vi "Sample Application.vi"() -> ()   [LabVIEW 2010]
doc: "This is a demo to understand how to use Solo Server and Instant PLUS for online license activation."
uses:
  C:/Program Files (x86)/SoftwareKey/Instant PLUS/IP2Lib32.dll
panel:
  in  "Upgrade to Ultimate":bool
  in  "Exit":bool
  in  "Deactviate":bool
  out "Activated Version":bool
  out "Demo  Version":bool
  out "AW Ultimate Mode":bool
  out "AW Ultra Mode":bool
  out "AW Omnia Mode":bool
  # "Sample Application"
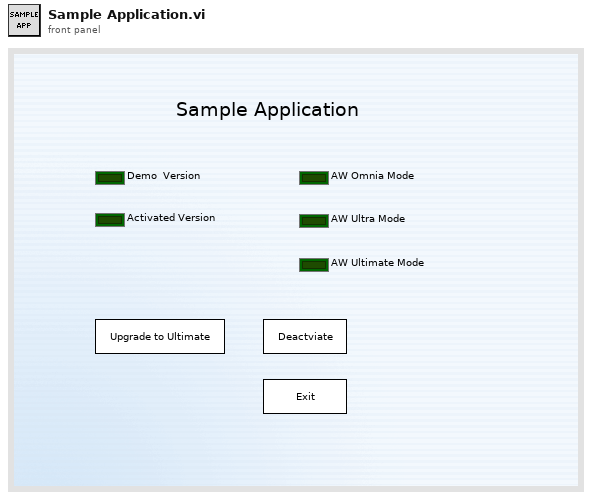
[diagram p1: front panel]
types:
  T1 = enum8{"Enabled", "Disabled", "Disabled and Grayed Out"}
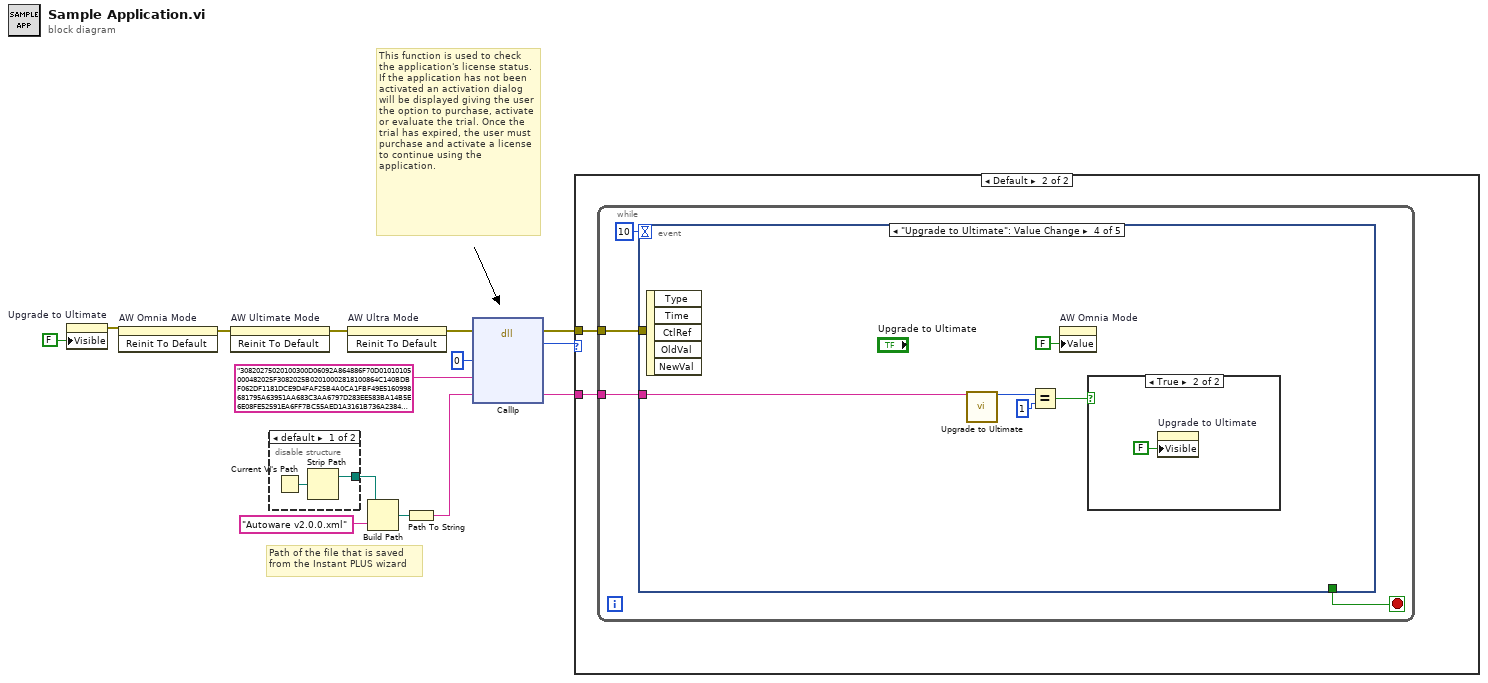
[diagram p0: block diagram]
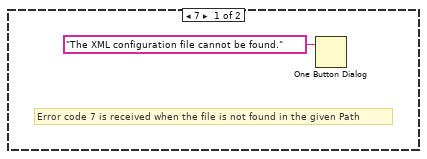
[diagram p2: hidden frame]
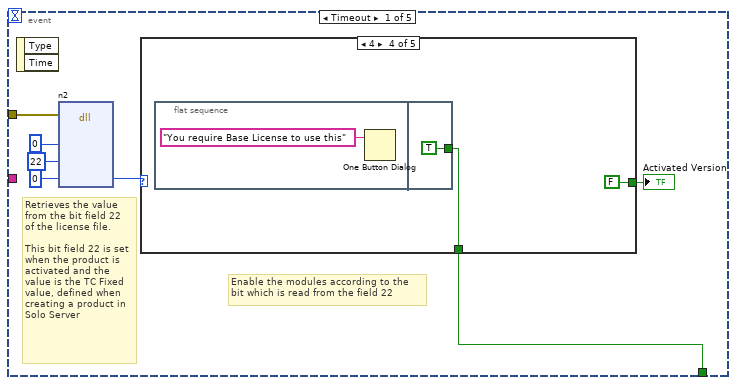
[diagram p3: hidden frame]
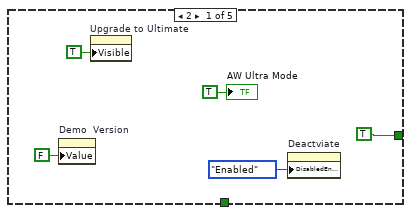
[diagram p4: hidden frame]
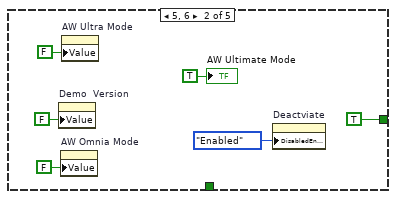
[diagram p5: hidden frame]
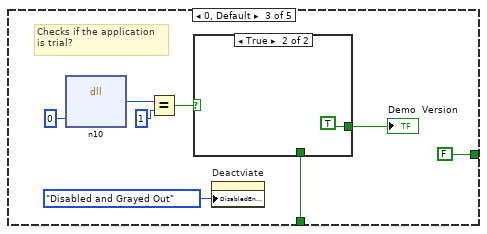
[diagram p6: hidden frame]
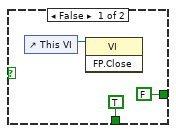
[diagram p7: hidden frame]
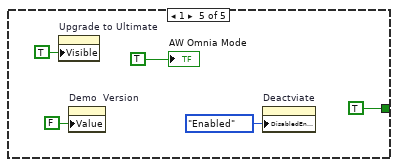
[diagram p8: hidden frame]
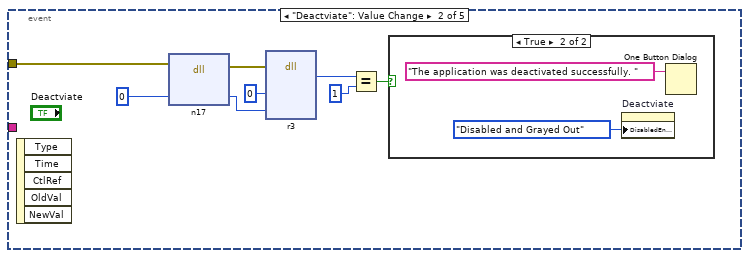
[diagram p9: hidden frame]
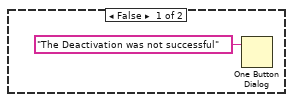
[diagram p10: hidden frame]
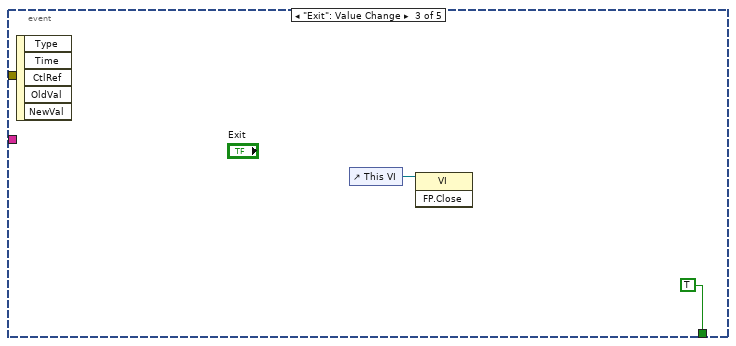
[diagram p11: hidden frame]
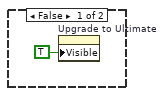
[diagram p12: hidden frame]
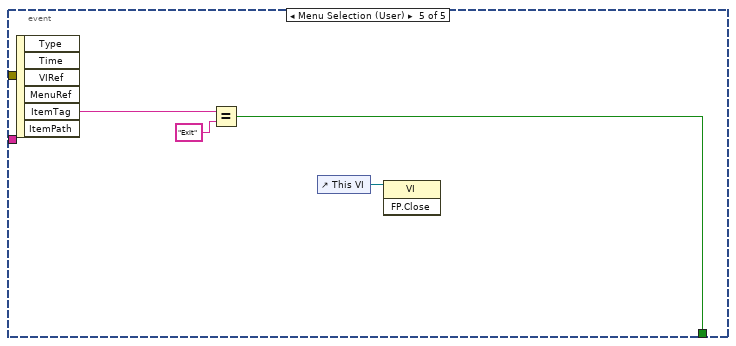
[diagram p13: hidden frame]
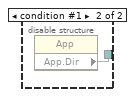
[diagram p14: hidden frame]
diagram:
  # "Path of the file that is saved \nfrom the Instant PLUS wizard"
  # "This function is used to check the application's license status. If the application has not been activated an activation dialog will be displayed giving the user the option to purchase, activate or evaluate the trial. Once the trial has expired, the user must purchase and activate a license to continue using the application."
  n1 = property on="Upgrade to Ultimate" class="Bool"("Visible"=FALSE) -> (error out=w3:errorcluster)  [unwired: 2 in, 1 out]
  n2 = invoke on="AW Omnia Mode" class="Bool (strict)" method="Reinit To Default"(error in=w3) -> (error out=w9:errorcluster)  [unwired: 2 in, 2 out]
  n3 = invoke on="AW Ultimate Mode" class="Bool (strict)" method="Reinit To Default"(error in=w9) -> (error out=w8:errorcluster)  [unwired: 2 in, 2 out]
  n4 = disable-structure shown="default" {
    disable-tunnel: [w16 w17] -> w2
    frame condition #0 (active) {
      n5 = Current VI's Path() -> (path=w15:path)
      n6 = Strip Path(path=w15) -> (stripped path=w16:path)  [unwired: 1 out]
    }
    frame condition #1 {
      n7 = property class="App"() -> ("App.Dir"=w17:path)  [unwired: 2 in, 2 out]
    }
  }
  n8 = invoke on="AW Ultra Mode" class="Bool (strict)" method="Reinit To Default"(error in=w8) -> (error out=w7:errorcluster)  [unwired: 2 in, 2 out]
  n9 = Build Path(base path=w2, name or relative path="Autoware v2.0.0.xml") -> (appended path=w13:path)
  n10 = Path To String(path=w13) -> (string=w14:string)
  n11 = dll-call lib="C:/Program Files (x86)/SoftwareKey/Instant PLUS/IP2Lib32.dll" fn="CallIp"(error in=w7, "flags"=0, "key"="30820275020100300D06092A864886F70D01010105000482025F3082025B02010002818100864C140BDBF062DF1181DCE9D4FAF25B4A0CA1FBF49E5160998681795A63951AA683C3AA6797D283EE583BA14B5E6E08FE52591EA6FF7BC55AED1A3161B736A2384D870C7207CC8E0C44F3FA09198B5C5B93A3664E7E03A0649458AD77C39D105654BF6D9AB9740C204A6EEE81CCFF07CA72CE9B1B6C7B6A51E0E7FB828A71050201110281802B72F76D3FA09875587CD687E305E4FF6AC7DA0DC0151A53F56F48019D3E55E2F9A319A81274E239BE0D7CB42EF8E75D4338C27ADBAD02657F4CB5A6908E193403A635934E3586225F27BF45D9C9E9ED9CFCFD5F08C52C6CFB1FB7415746DD7D51C4C534D770EAAE174BC1FFC315035FFAA70DEA8A613053DEEFD2921B82A04302...", "path"=w14) -> (error out=w5:errorcluster, "result"=w6:i32, "path"=w1:string)  [unwired: 4 in, 1 out]
  n12 = case shown="Default" w6 {
    tunnel: w5 -> [_ w20]
    tunnel: w1 -> [_ w19]
    frame 7 {
      # "Error code 7 is received when the file is not found in the given Path"
      n13 = One Button Dialog(message="The XML configuration file cannot be found.") -> ()  [unwired: 1 in, 1 out]
    }
    frame Default {
      n14 = while {
        tunnel: w20 -> [w22]
        tunnel: w19 -> [w21]
        stop <- w23 stop-if-true
        n15 = event shown="[3] \"Upgrade to Ultimate\": Value Change" {
          selector: _ -> [_ _ _ _ _]
          dyn-events: _ -> [_ _ _ _ _]
          timeout: 10 -> [_ _ _ _ _]
          tunnel: [w30 _ TRUE ("Exit") _ w85] -> w23
          tunnel: w22 -> [w25 w67 _ _ _]
          tunnel: w21 -> [_ _ _ w77 _]
          event Timeout {
            # "Enable the modules according to the\nbit which is read from the field 22"
            # "Retrieves the value\nfrom the bit field 22\nof the license file.\n\nThis bit field 22 is set\nwhen the product is \nactivated and the \nvalue is the TC Fixed \nvalue, defined when\ncreating a product in\nSolo Server"
            n16 = event-data() -> ()  [unwired: 1 in, 2 out]
            n17 = dll-call lib="C:/Program Files (x86)/SoftwareKey/Instant PLUS/IP2Lib32.dll" fn="n2"(error in=w25, "flags"=0, "varno"=22, "value"=0) -> ("value"=w26:i32)  [unwired: 5 in, 2 out]
            n18 = case shown="4" w26 {
              tunnel: [TRUE ("AW Ultra Mode") TRUE ("AW Ultra Mode") FALSE ("AW Ultra Mode") FALSE ("AW Ultra Mode") TRUE ("AW Ultra Mode")] -> w31
              tunnel: [_ _ w43 w55 _] -> w30
              frame 2 {
                n19 = property on="Demo  Version" class="Bool (strict)"("Value"=FALSE ("Demo  Version")) -> ()  [unwired: 2 in, 2 out]
                n20 = property on="Upgrade to Ultimate" class="Bool"("Visible"=TRUE) -> ()  [unwired: 2 in, 2 out]
                n21 = property on="Deactviate" class="Bool"("DisabledEnum"=T1."Enabled" ("Disabled")) -> ()  [unwired: 2 in, 2 out]
                "AW Ultra Mode" <- TRUE ("AW Ultra Mode")
              }
              frame 5, 6 {
                n22 = property on="Demo  Version" class="Bool (strict)"("Value"=FALSE ("Demo  Version")) -> ()  [unwired: 2 in, 2 out]
                n23 = property on="AW Omnia Mode" class="Bool (strict)"("Value"=FALSE ("AW Omnia Mode")) -> ()  [unwired: 2 in, 2 out]
                n24 = property on="AW Ultra Mode" class="Bool (strict)"("Value"=FALSE ("AW Ultra Mode")) -> ()  [unwired: 2 in, 2 out]
                n25 = property on="Deactviate" class="Bool"("DisabledEnum"=T1."Enabled" ("Disabled")) -> ()  [unwired: 2 in, 2 out]
                "AW Ultimate Mode" <- TRUE ("AW Ultimate Mode")
              }
              frame 0, Default {
                # "Checks if the application\nis trial?"
                n26 = dll-call lib="C:/Program Files (x86)/SoftwareKey/Instant PLUS/IP2Lib32.dll" fn="n10"("flags"=0) -> ("result"=w47:i32)  [unwired: 4 in, 2 out]
                n27 = Equal?(x=w47, y=1) -> (x = y?=w45:bool)
                n28 = case shown="True" w45 {
                  tunnel: [FALSE ("Demo  Version") TRUE ("Demo  Version")] -> w44
                  tunnel: [TRUE ("Demo  Version") _] -> w43
                  frame False {
                    n29 = control-ref of="This VI"() -> (w51:refnum<vi>)
                    n30 = invoke class="VI" method="FP.Close"(reference=w51) -> ()  [unwired: 2 in, 3 out]
                  }
                  frame True {
                  }
                }
                "Demo  Version" <- w44
                n31 = property on="Deactviate" class="Bool"("DisabledEnum"=T1."Disabled and Grayed Out" ("Disabled")) -> ()  [unwired: 2 in, 2 out]
              }
              frame 4 {
                n32 = flat-sequence {
                  tunnel: [TRUE ("Demo  Version")] -> w55
                  frame #0 {
                    n33 = One Button Dialog(message="You require Base License to use this") -> ()  [unwired: 1 in, 1 out]
                  }
                  frame #1 {
                  }
                }
              }
              frame 1 {
                n34 = property on="Upgrade to Ultimate" class="Bool"("Visible"=TRUE) -> ()  [unwired: 2 in, 2 out]
                n35 = property on="Demo  Version" class="Bool (strict)"("Value"=FALSE ("Demo  Version")) -> ()  [unwired: 2 in, 2 out]
                n36 = property on="Deactviate" class="Bool"("DisabledEnum"=T1."Enabled" ("Disabled")) -> ()  [unwired: 2 in, 2 out]
                "AW Omnia Mode" <- TRUE ("AW Omnia Mode")
              }
            }
            "Activated Version" <- w31
          }
          event "Deactviate": Value Change {
            n37 = event-data() -> ()  [unwired: 1 in, 5 out]
            n38 = dll-call lib="C:/Program Files (x86)/SoftwareKey/Instant PLUS/IP2Lib32.dll" fn="n17"(error in=w67, "handle"=0) -> (error out=w66:errorcluster, "handle"=w65:i32)  [unwired: 3 in, 1 out]
            n39 = dll-call lib="C:/Program Files (x86)/SoftwareKey/Instant PLUS/IP2Lib32.dll" fn="r3"(error in=w66, "flags"=0, "handle"=w65) -> ("result"=w70:i32)  [unwired: 4 in, 2 out]
            n40 = Equal?(x=w70, y=1) -> (x = y?=w68:bool)
            n41 = case shown="True" w68 {
              frame False {
                n42 = One Button Dialog(message="The Deactivation was not successful") -> ()  [unwired: 1 in, 1 out]
              }
              frame True {
                n43 = property on="Deactviate" class="Bool"("DisabledEnum"=T1."Disabled and Grayed Out" ("Disabled")) -> ()  [unwired: 2 in, 2 out]
                n44 = One Button Dialog(message="The application was deactivated successfully. ") -> ()  [unwired: 1 in, 1 out]
              }
            }
          }
          event "Exit": Value Change {
            n45 = event-data() -> ()  [unwired: 1 in, 5 out]
            n46 = control-ref of="This VI"() -> (w75:refnum<vi>)
            n47 = invoke class="VI" method="FP.Close"(reference=w75) -> ()  [unwired: 2 in, 3 out]
          }
          event "Upgrade to Ultimate": Value Change {
            n48 = event-data() -> ()  [unwired: 1 in, 5 out]
            n49 = call "Upgrade to Ultimate.vi"("path"=w77) -> ("result"=w80:i32)  [unwired: 14 in]
            n50 = Equal?(x=w80, y=1) -> (x = y?=w78:bool)
            n51 = property on="AW Omnia Mode" class="Bool (strict)"("Value"=FALSE ("AW Omnia Mode")) -> ()  [unwired: 2 in, 2 out]
            n52 = case shown="True" w78 {
              frame False {
                n53 = property on="Upgrade to Ultimate" class="Bool"("Visible"=TRUE) -> ()  [unwired: 2 in, 2 out]
              }
              frame True {
                n54 = property on="Upgrade to Ultimate" class="Bool"("Visible"=FALSE) -> ()  [unwired: 2 in, 2 out]
              }
            }
          }
          event Menu Selection (User) {
            n55 = event-data() -> ("ItemTag"=w87:string)  [unwired: 1 in, 5 out]
            n56 = Equal?(x=w87, y="Exit") -> (x = y?=w85:bool)
            n57 = control-ref of="This VI"() -> (w84:refnum<vi>)
            n58 = invoke class="VI" method="FP.Close"(reference=w84) -> ()  [unwired: 2 in, 3 out]
          }
        }
      }
    }
  }
